vi "Get Full Help.vi"(8 "error in (no error)":errorcluster, 11 "Update in":refnum<class "Update.lvclass">) -> (0 "error out":errorcluster, 2 "Full Help":string, 3 "Update out":refnum<class "Update.lvclass">)   [LabVIEW 2020, in "Update.lvlib" / "Update.lvclass"]
uses:
  Update.lvclass
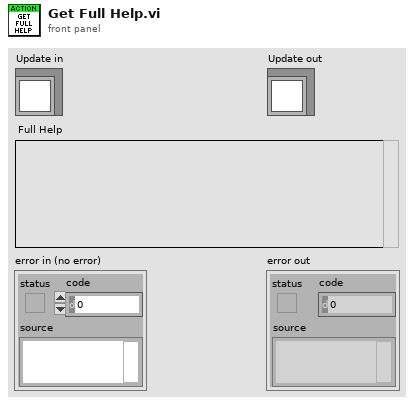
[diagram p1: front panel]
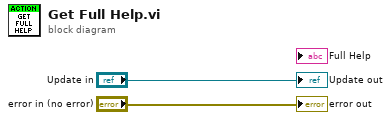
[diagram p0: block diagram]
diagram:
  "error out" <- "error in (no error)"
  "Update out" <- "Update in"
